vi "gxml_Error74.vi"(5 "error in (no error)":errorcluster) -> (2 "error out":errorcluster)   [LabVIEW 2011, in "Third Party VIs.lvlib" / "GXML.lvlib"]
uses:
  GXML.lvlib
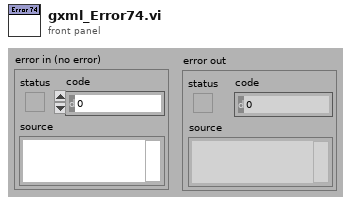
[diagram p1: front panel]
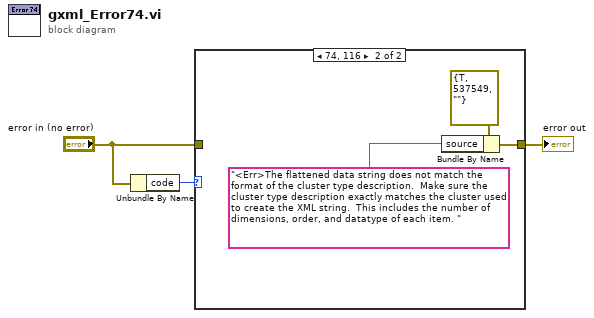
[diagram p0: block diagram]
diagram:
  n1 = Unbundle By Name("error in (no error)") -> ("code"=w1:i32)
  n2 = case shown="74, 116" w1 {
    tunnel: "error in (no error)" -> [w4 _]
    tunnel: [w4 w6] -> w2
    frame 0, Default {
    }
    frame 74, 116 {
      n3 = Bundle By Name(cluster=errorcluster {"status"=TRUE, "code"=537549, "source"=""} ("error in"), "source"="<Err>The flattened data string does not match the format of the cluster type description.  Make sure the cluster type description exactly matches the cluster used to create the XML string.  This includes the number of dimensions, order, and datatype of each item. ") -> (w6:errorcluster)
    }
  }
  "error out" <- w2
